vi "niScope Cal Adjust Frequency Response.vi"(0 "instrument handle":refnum<k15>, 5 "channels":string, 7 "range (V)":dbl format="%.2f", 9 "stimulus amplitude":dbl format="%.2f", 11 "error in":errorcluster, 12 "stimulus frequency":dbl format="%.2f") -> (4 "instrument handle out":refnum<k15>, 15 "error out":errorcluster)   [LabVIEW 2011]
doc: "For the NI 5622, calibrates the frequency response of the device. The VI is called multiple times, one for each frequency point in the sweep. The user must supply the <B>stimulus frequency</B> in hertz and <B>stimulus amplitude</B> in volts of the input signal."
uses:
  niScope_32.dll
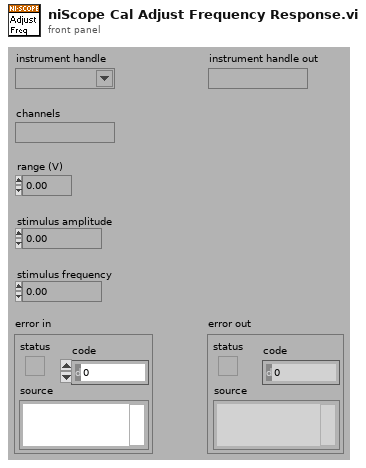
[diagram p1: front panel]
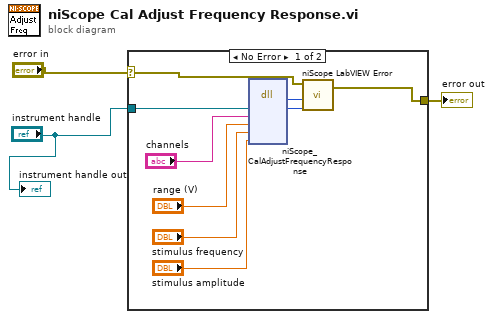
[diagram p0: block diagram]
diagram:
  n1 = case shown="No Error" "error in" {
    selector: "error in" -> [w6 w13]
    tunnel: [w7 w13] -> w3
    tunnel: "instrument handle" -> [w12 _]
    frame No Error {
      n2 = dll-call lib="niScope_*.*" fn="niScope_CalAdjustFrequencyResponse"("instrument handle"=w12, "Channel Name"="channels", "range"="range (V)", "stimulusFrequency"="stimulus frequency", "stimulusAmplitude"="stimulus amplitude") -> ("status"=w8:i32, "instrument handle"=w9:u32)  [unwired: 7 in, 2 out]
      n3 = call <instrlib>:"niScope LabVIEW Error.vi"("instrument handle"=w9, "niScope error code (0)"=w8, "error in (no error)"=w6) -> ("error out"=w7:errorcluster)  [unwired: 2 in]
    }
    frame Error {
    }
  }
  "error out" <- w3
  "instrument handle out" <- "instrument handle"
